vi "SimpleCMDwithSnapshot.vi"(6 "Dest Format":string(combo)="{6fddc324-4e03-4bfe-b185-3d77768dc90e}", 7 "HTTP_address":string, 10 "Value":T3, 11 "Refnum in":T2) -> (3 "headers":string)   [LabVIEW 2016]
uses:
  cgi_string.ctl
  <vilib>/httpClient/ClientHandle.ctl
  <vilib>/vision/Image Controls.llb/IMAQ Image.ctl
  <vilib>/httpClient/LabVIEWHTTPClient.lvlib
panel:
  out "Dest Format":string(combo)="{6fddc324-4e03-4bfe-b185-3d77768dc90e}"
  out "Image":T1(plugin-control)
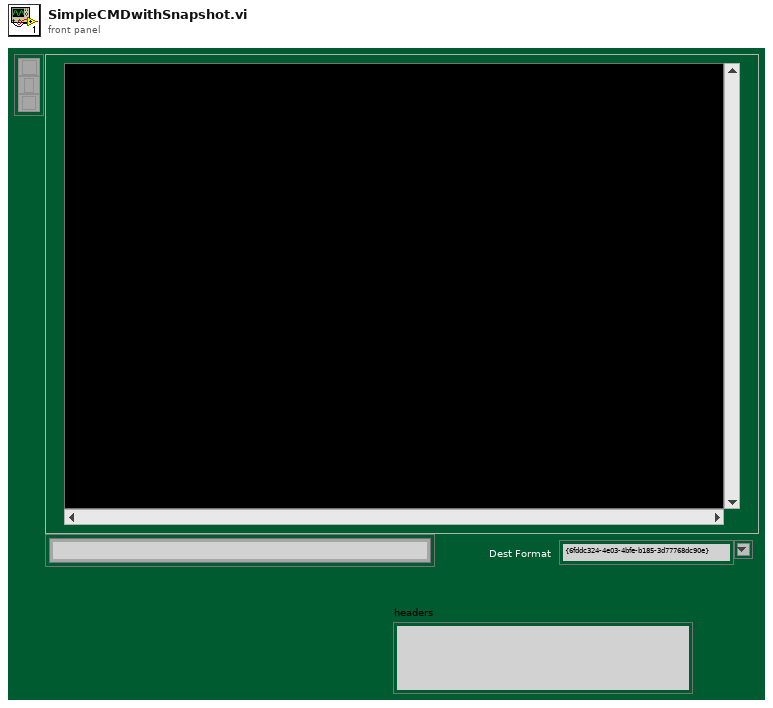
[diagram p1: front panel]
types:
  T1 = typedef "IMAQ Image.ctl" = refnum<image>
  T2 = typedef "LabVIEWHTTPClient.lvlib/ClientHandle.ctl" = refnum<k1>
  T3 = typedef "cgi_string.ctl" = string
  T4 = typedef "Image Type" = u32
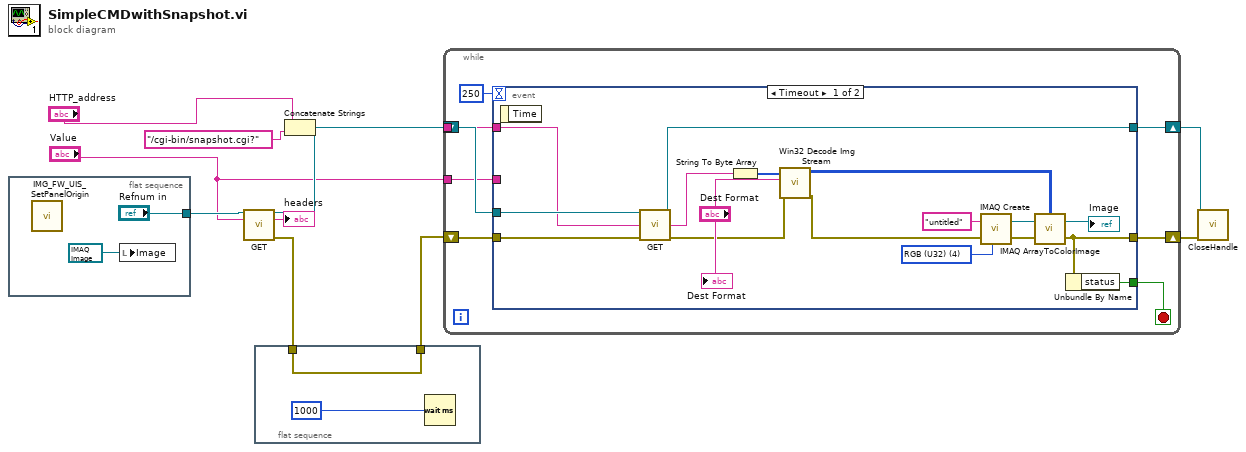
[diagram p0: block diagram]
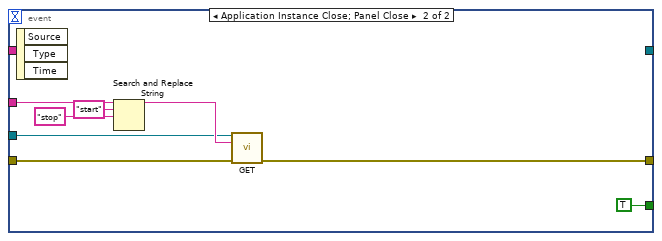
[diagram p2: hidden frame]
diagram:
  n1 = flat-sequence {
    tunnel: ["Refnum in"] -> w11
    frame #0 {
      n2 = call "IMG_FW_UIS_SetPanelOrigin.vi"() -> ()  [unwired: 11 in, 1 out]
      n3 = local write "Image"(T1 refnum ("New Image")) -> ()
    }
  }
  n4 = call <vilib>:"GET.vi"("client handle"=w11, "url"="Value") -> ("client handle out"=w9:T2, "headers"=→"headers":string, "error out"=w4:errorcluster)  [unwired: 10 in, 1 out]
  n5 = flat-sequence {
    tunnel: [w15] -> w3
    tunnel: w4 -> [w15]
    frame #0 {
      n6 = Wait (ms)(milliseconds to wait=u32 1000) -> ()  [unwired: 1 out]
    }
  }
  n7 = Concatenate Strings("HTTP_address", "/cgi-bin/snapshot.cgi?") -> (w5:string)
  n8 = while {
    tunnel: w5 -> [w20]
    shift-right: [w21] -> w8
    shift-left: w9 -> [w22]
    shift-right: [w23] -> w10
    shift-left: w3 -> [w19]
    tunnel: "Value" -> [w16]
    stop <- w17 stop-if-true
    n9 = event shown="[0] Timeout" {
      selector: _ -> [_ _]
      dyn-events: _ -> [_ _]
      timeout: 250 -> [_ _]
      tunnel: [w25 w41] -> w23
      tunnel: w22 -> [w30 w43]
      tunnel: [w29 _] -> w21
      tunnel: w20 -> [w27 _]
      tunnel: w19 -> [w26 w42]
      tunnel: [w24 TRUE] -> w17
      tunnel: w16 -> [_ w47]
      event Timeout {
        w39 = T4 4 items=["Grayscale (U8)", "Grayscale (I16)", "Grayscale (SGL)", "Complex (CSG)", "RGB (U32)", "HSL (U32)", "RGB (U64)", "Grayscale (U16)"] ("Image Type")
        n10 = event-data() -> ()  [unwired: 1 in, 1 out]
        n11 = call <vilib>:"GET.vi"("client handle"=w30, "url"=w27, "error in (no error)"=w26) -> ("client handle out"=w29:T2, "body"=w31:string, "error out"=w28:errorcluster)  [unwired: 9 in, 1 out]
        n12 = String To Byte Array(string=w31) -> (unsigned byte array=w37:u8[])
        n13 = call "Win32 Decode Img Stream.vi"("error in (no error)"=w28, "Dest Format"="Dest Format", "Image Data"=w37) -> ("error out"=w34:errorcluster, "Dest"=w36:u32[][])  [unwired: 4 in, 3 out]
        n14 = call "IMAQ Create"("Image Name"="untitled", "Image Type"=w39, "error in (no error)"=w34) -> ("New Image"=w40:T1, "error out"=w35:errorcluster)  [unwired: 2 in]
        n15 = call "IMAQ ArrayToColorImage"("Image Pixels (U32)"=w36, "Image"=w40, "error in (no error)"=w35) -> ("Image Out"=→"Image":T1, "error out"=w25:errorcluster)  [unwired: 2 in]
        n16 = Unbundle By Name(w25) -> ("status"=w24:bool)
        "Dest Format" <- "Dest Format"
      }
      event Application Instance Close; Panel Close {
        n17 = event-data() -> ()  [unwired: 1 in, 3 out]
        n18 = Search and Replace String(input string=w47, search string="start", replace string="stop" ("replace string (\"\")")) -> (result string=w44:string)  [unwired: 5 in, 3 out]
        n19 = call <vilib>:"GET.vi"("client handle"=w43, "url"=w44, "error in (no error)"=w42) -> ("error out"=w41:errorcluster)  [unwired: 9 in, 3 out]
      }
    }
  }
  n20 = call <vilib>:"CloseHandle.vi"("client handle"=w8, "error in (no error)"=w10) -> ()  [unwired: 13 in, 1 out]
